vi "Calculate Heading Components.vi"(11 "Heading In [deg]":sgl) -> (2 "Sin Heading":sgl, 3 "Cos Heading":sgl)   [LabVIEW 2015, in "Motion.lvclass"]
uses:
  Motion.lvclass
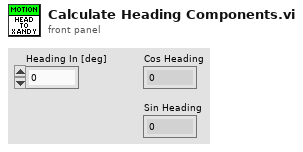
[diagram p1: front panel]
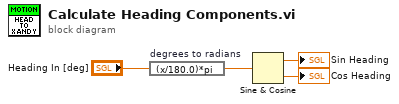
[diagram p0: block diagram]
diagram:
  n1 = expression code="(x/180.0)*pi" "degrees to radians"("Heading In [deg]") -> (w2:sgl)
  n2 = Sine & Cosine(0:w2) -> (1:→"Sin Heading":sgl, 2:→"Cos Heading":sgl)
